vi "Read_from_motor_log_file.vi"(11 "File name in":path) -> (0 "subarray":dbl[](array[numeric]), 1 "Number of steps total":dbl, 2 "all rows":dbl[][](array[numeric]) format="%0.3f", 3 "File name out":path, 4 "Number of steps directional":dbl, 5 "Cycle number":dbl)   [LabVIEW 2012]
uses:
  <vilib>/Utility/file.llb/Read From Spreadsheet File (DBL).vi
panel:
  in  "error in":errorcluster
  out "error out":errorcluster
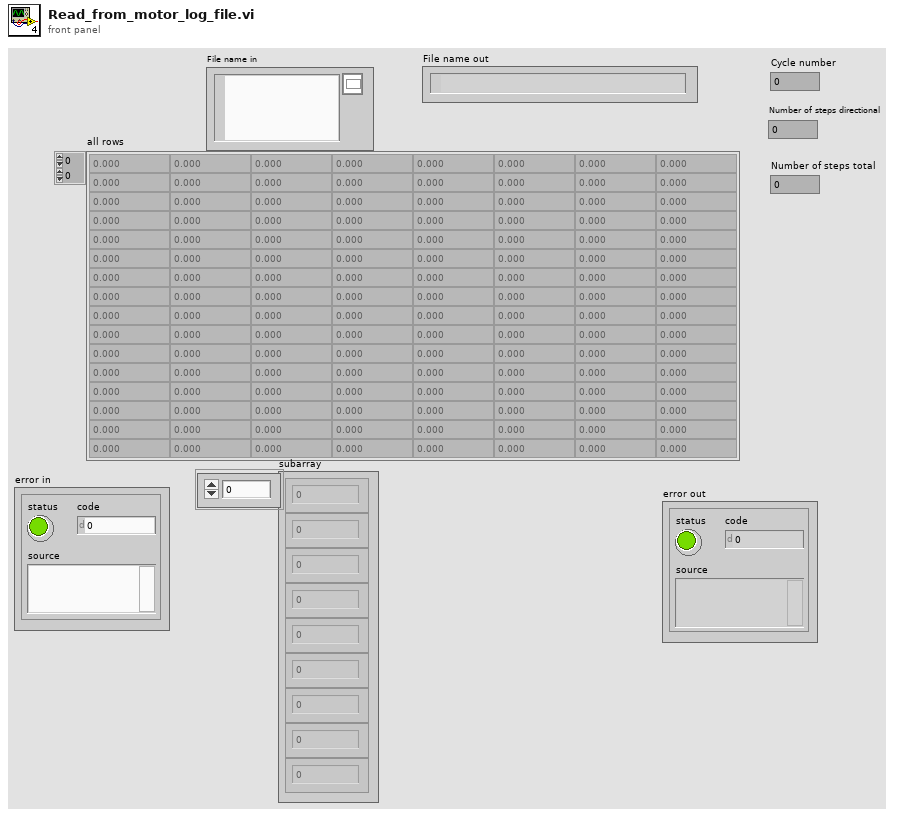
[diagram p1: front panel]
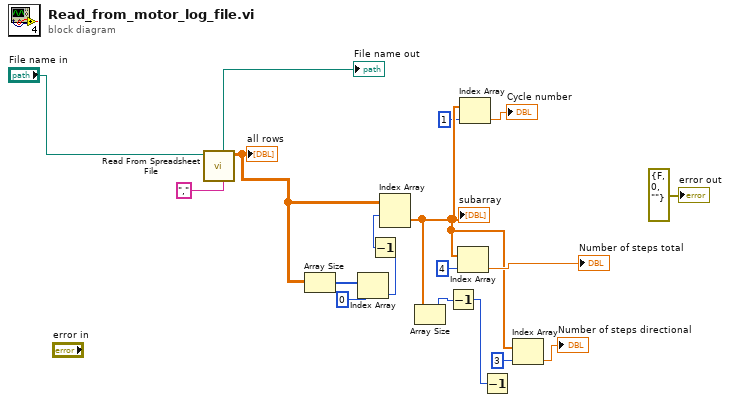
[diagram p0: block diagram]
diagram:
  n1 = call-poly <vilib>:"Read From Spreadsheet File.vi"("delimiter (\\t)"="," ("delimiter (\\t)"), "file path (dialog if empty)"="File name in") -> ("all rows"=w15:dbl[][], "new file path (Not A Path if cancelled)"=→"File name out":path)  [unwired: 5 in, 3 out]
  "all rows" <- w15
  n2 = Array Size(array=w15) -> (size(s)=w14:i32[])
  n3 = Index Array(array=w14, index=0) -> (element=w12:i32)
  n4 = Decrement(x=w12) -> (x-1=w11:i32)
  n5 = Index Array(array=w15, index (row)=w11) -> (element=w5:dbl[])  [unwired: 1 in]
  "subarray" <- w5
  n6 = Array Size(array=w5) -> (size(s)=w7:i32)
  n7 = Decrement(x=w7) -> (x-1=w6:i32)
  n8 = Index Array(array=w5, index=4) -> (element=→"Number of steps total":dbl)
  n9 = Index Array(array=w5, index=1) -> (element=→"Cycle number":dbl)
  n10 = Decrement(x=w6) -> ()  [unwired: 1 out]
  n11 = Index Array(array=w5, index=3) -> (element=→"Number of steps directional":dbl)
  "error out" <- errorcluster {"status"=FALSE, "code"=0, "source"=""} ("error out")
